vi "Draw_Pattern_exercise_ms.vi"() -> ()   [LabVIEW 2016]
uses:
  Classes/Controller/Motion/A3200 Folder/A3200.lvclass
panel:
  out "XYZTheta Out 2":dbl[](array[numeric])
  out "XYZTheta Out":dbl[](array[numeric])
  in  "Speed":dbl
  out "subarray":dbl[](array[numeric])
  in  "d_y":dbl
  in  "d_x":dbl
  out "element":i32
  out "Array":dbl[][](array[numeric])
  in  "O_y":dbl
  in  "O_x":dbl
  in  "P_num":i32
  in  "start":bool
  in  "stop":bool
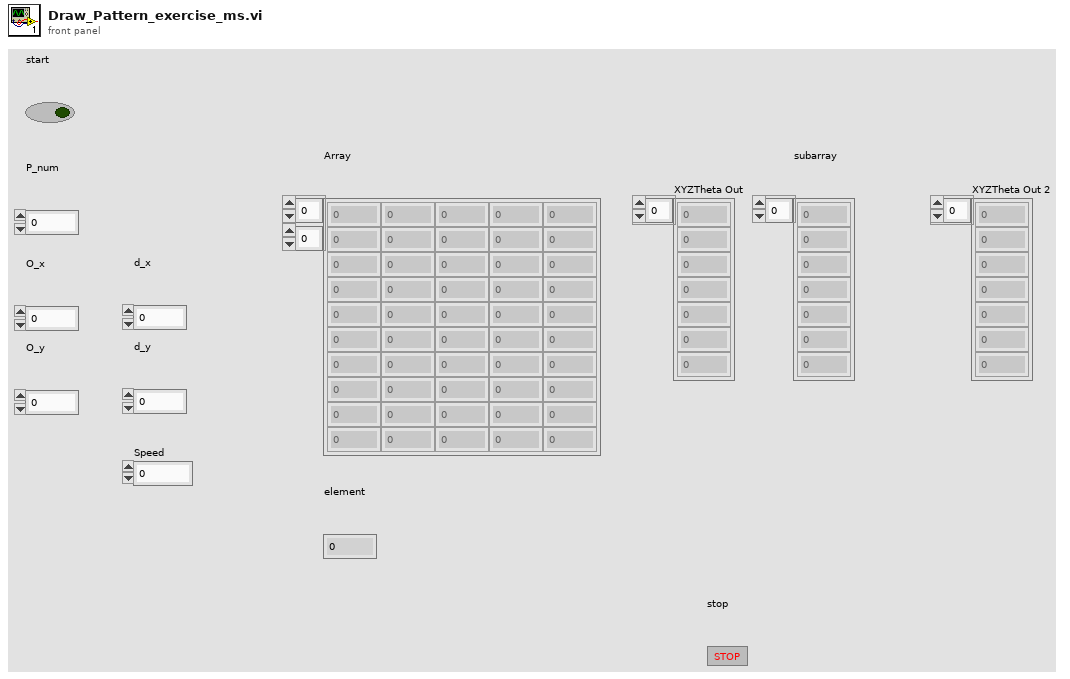
[diagram p1: front panel]
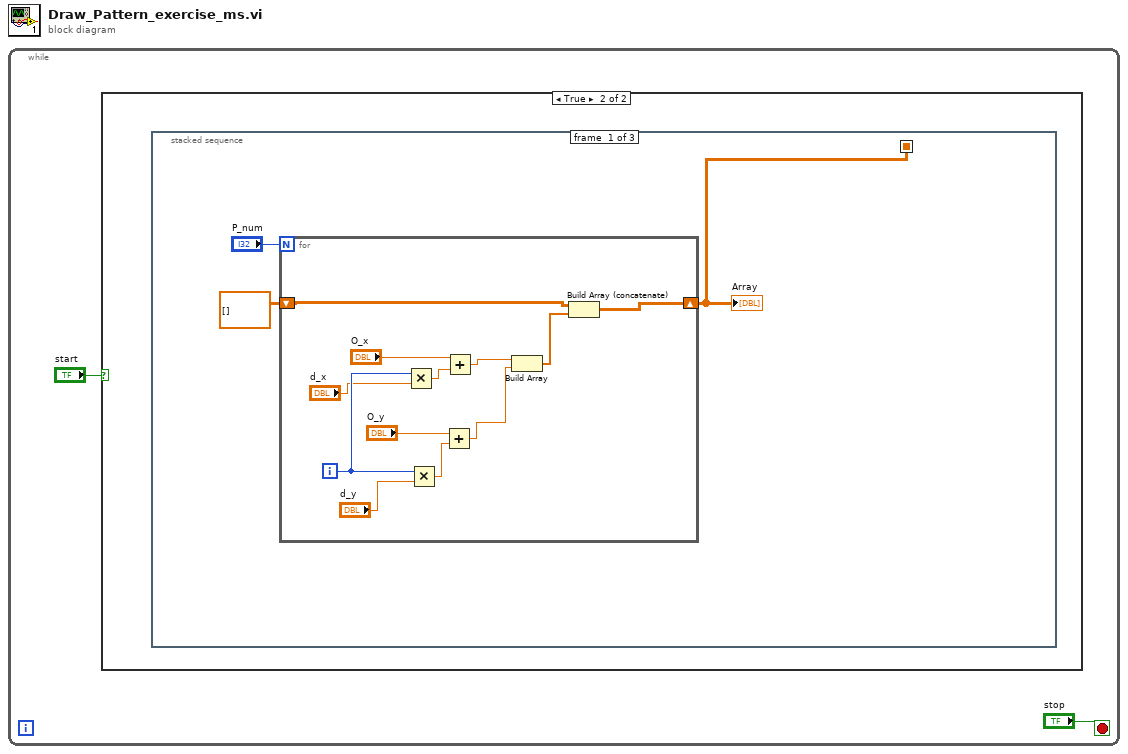
[diagram p0: block diagram]
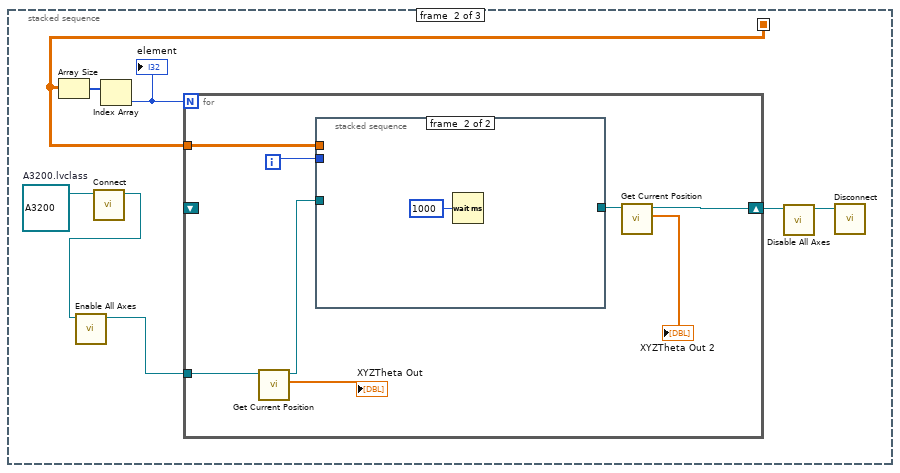
[diagram p3: hidden frame]
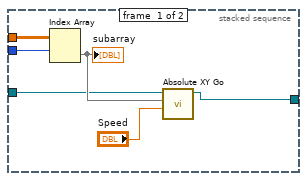
[diagram p4: hidden frame]
diagram:
  n1 = while {
    stop <- "stop" stop-if-true
    n2 = case shown="True" "start" {
      frame False {
      }
      frame True {
        n3 = stacked-sequence {
          seq-local: [w4 _ _] -> [_ w23 _]
          frame #0 {
            n4 = for {
              N: "P_num" -> [_]
              shift-right: [w9] -> w4
              shift-left: dbl[][] [] -> [w8]
              i -> [w13]
              n5 = Multiply(x=w13, y="d_x") -> (x*y=w14:dbl)
              n6 = Multiply(x=w13, y="d_y") -> (x*y=w17:dbl)
              n7 = Add(x="O_y", y=w17) -> (x+y=w11:dbl)
              n8 = Add(x="O_x", y=w14) -> (x+y=w12:dbl)
              n9 = Build Array(w12, w11) -> (w10:dbl[])
              n10 = Build Array (concatenate)(w8, w10) -> (w9:dbl[][])
            }
            "Array" <- w4
          }
          frame #1 {
            w22 = refnum<class "A3200.lvclass"> refnum  # A3200.lvclass
            n11 = Array Size(array=w23) -> (size(s)=w25:i32[])
            n12 = call-dynamic "Connect.vi"("Gantry in"=w22) -> ("Gantry out"=w20:refnum<class "A3200.lvclass">)  [unwired: 9 in, 1 out]
            n13 = call-dynamic "Enable All Axes.vi"("A3200 in"=w20) -> ("A3200 out"=w21:refnum<class "A3200.lvclass">)  [unwired: 9 in, 1 out]
            n14 = Index Array(array=w25) -> (element=w24:i32)  [unwired: 1 in]
            "element" <- w24
            n15 = for {
              N: w24 -> [_]
              tunnel: w23 -> [w33]
              tunnel: w21 -> [w31]
              shift-right: [w26] -> w18
              shift-left: _ -> [_]
              i -> [w32]
              n16 = call-dynamic "Get Current Position.vi"("Gantry in"=w31) -> ("XYZTheta Out"=→"XYZTheta Out":dbl[], "Gantry out"=w30:refnum<class "A3200.lvclass">)  [unwired: 8 in, 1 out]
              n17 = stacked-sequence {
                tunnel: w33 -> [w39 _]
                tunnel: w32 -> [w38 _]
                tunnel: w30 -> [w35 _]
                tunnel: [w34 _] -> w28
                frame #0 {
                  n18 = Index Array(array=w39, index (row)=w38) -> (element=w37:dbl[])  [unwired: 1 in]
                  "subarray" <- w37
                  n19 = call-dynamic "Absolute XY Go.vi"("Speed"="Speed", "XY"=w37, "Gantry in"=w35) -> ("Gantry out"=w34:refnum<class "A3200.lvclass">)  [unwired: 7 in, 1 out]
                }
                frame #1 {
                  n20 = Wait (ms)(milliseconds to wait=u32 1000) -> ()  [unwired: 1 out]
                }
              }
              n21 = call-dynamic "Get Current Position.vi"("Gantry in"=w28) -> ("XYZTheta Out"=→"XYZTheta Out 2":dbl[], "Gantry out"=w26:refnum<class "A3200.lvclass">)  [unwired: 8 in, 1 out]
            }
            n22 = call-dynamic "Disable All Axes.vi"("Gantry in"=w18) -> ("Gantry out"=w19:refnum<class "A3200.lvclass">)  [unwired: 9 in, 1 out]
            n23 = call-dynamic "Disconnect.vi"("Gantry in"=w19) -> ()  [unwired: 9 in, 1 out]
          }
          frame #2 {
          }
        }
      }
    }
  }
